vi "LanchHistgramWin.vi"(8 "error in (no error)":errorcluster, 11 "DisplayerUI in":refnum<class "DisplayerUI.lvclass">) -> (0 "error out":errorcluster, 3 "DisplayerUI out":refnum<class "DisplayerUI.lvclass">)   [LabVIEW 2020, in "DisplayerUI.lvlib" / "DisplayerUI.lvclass"]
uses:
  DisplayerUI.lvclass
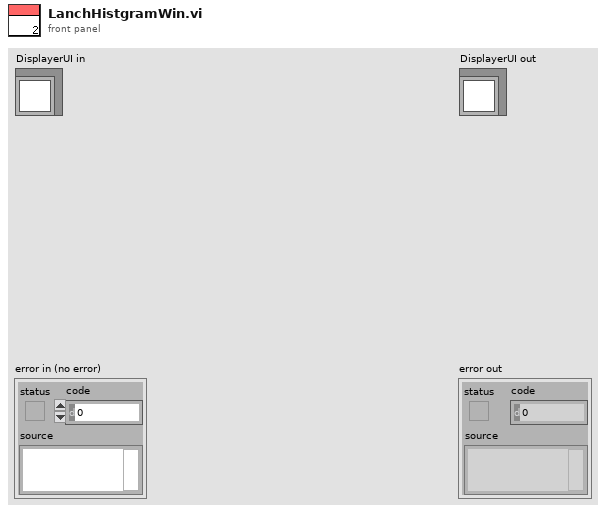
[diagram p1: front panel]
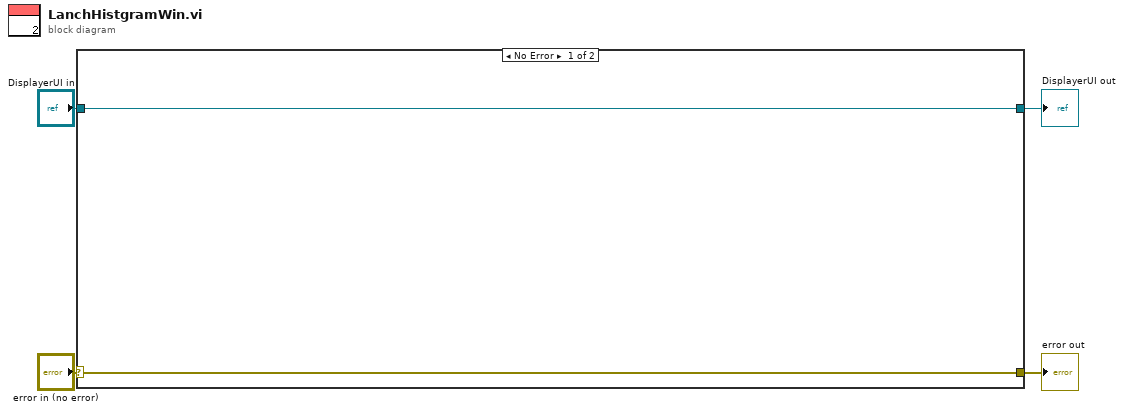
[diagram p0: block diagram]
diagram:
  n1 = case shown="No Error" "error in (no error)" {
    selector: "error in (no error)" -> [w6 w8]
    tunnel: [w6 w8] -> w3
    tunnel: [w5 w7] -> w1
    tunnel: "DisplayerUI in" -> [w5 w7]
    frame No Error {
    }
    frame Error {
    }
  }
  "error out" <- w3
  "DisplayerUI out" <- w1
